vi "Multiplexer(four-One).vi"() -> ()   [LabVIEW 2019]
panel:
  out "Result":bool
  in  "Toggle Switch Two":bool
  in  "Toggle Switch One":bool
  in  "Input Four":bool
  in  "Input Three":bool
  in  "Input Two":bool
  in  "Input One":bool
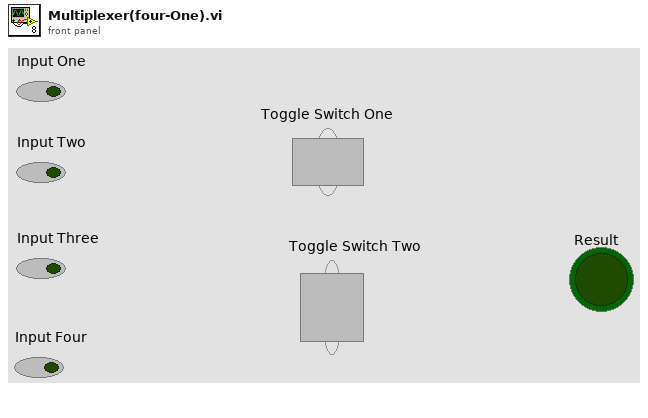
[diagram p1: front panel]
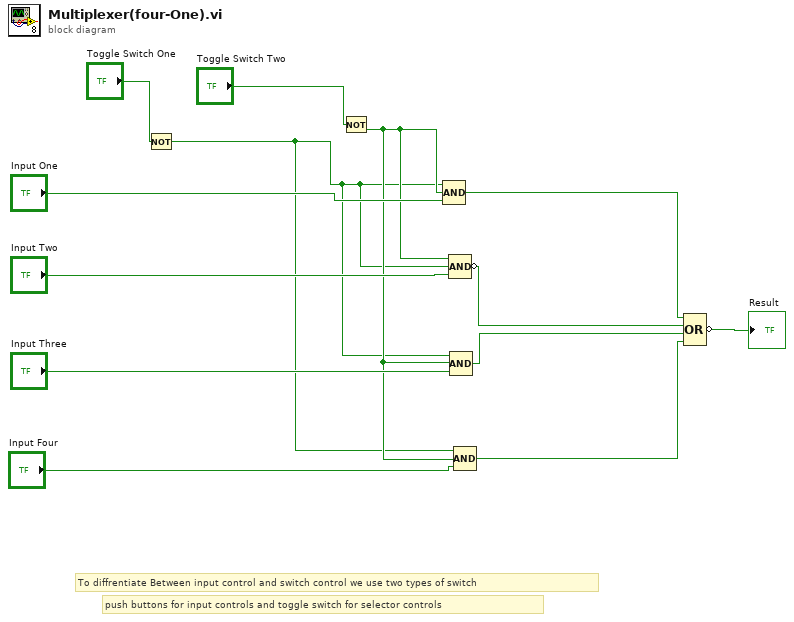
[diagram p0: block diagram]
diagram:
  # "push buttons for input controls and toggle switch for selector controls"
  # "To diffrentiate Between input control and switch control we use two types of switch"
  n1 = Not(x="Toggle Switch One") -> (.not. x?=w6:bool)
  n2 = Not(x="Toggle Switch Two") -> (.not. x?=w7:bool)
  n3 = Compound Arithmetic op=AND(w6, w7, "Input One") -> (w5:bool)
  n4 = Compound Arithmetic op=AND(w7, w6, "Input Two") -> (invert w4:bool)
  n5 = Compound Arithmetic op=AND(w6, w7, "Input Three") -> (w3:bool)
  n6 = Compound Arithmetic op=AND(w6, w7, "Input Four") -> (w2:bool)
  n7 = Compound Arithmetic op=OR(w5, w4, w3, w2) -> (invert →"Result":bool)
